vi "区域判断 - 副本.vi"(4 "压力数组":dbl[](array[numeric]), 5 "位移数组":dbl[](array[numeric]), 8 "区域最大位移":dbl, 9 "区域最小位移":dbl) -> (2 "区域最大压力":dbl=10000.0, 3 "区域最小压力":dbl)   [LabVIEW 2013]
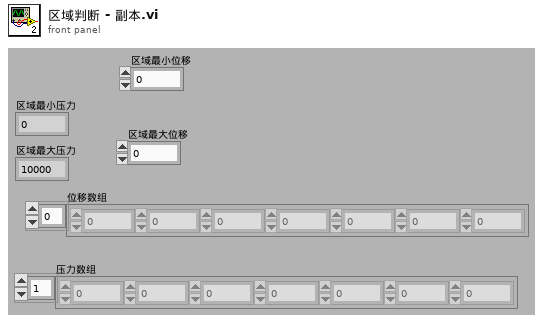
[diagram p1: front panel]
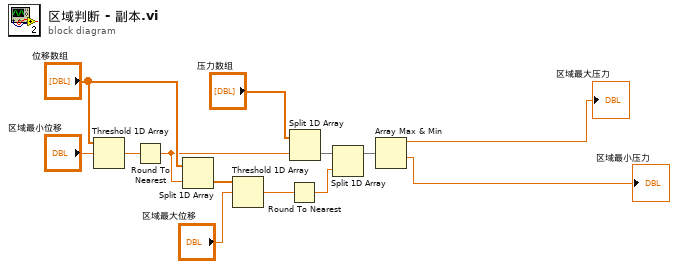
[diagram p0: block diagram]
diagram:
  n1 = Threshold 1D Array(2:"区域最小位移", 3:"位移数组") -> (0:w11:dbl)  [unwired: 1 in]
  n2 = Round To Nearest(number=w11) -> (nearest integer value=w6:dbl)
  n3 = Split 1D Array(array="位移数组", index=w6) -> (second subarray=w7:dbl[])  [unwired: 1 out]
  n4 = Threshold 1D Array(2:"区域最大位移", 3:w7) -> (0:w10:dbl)  [unwired: 1 in]
  n5 = Round To Nearest(number=w10) -> (nearest integer value=w4:dbl)
  n6 = Split 1D Array(array="压力数组", index=w6) -> (second subarray=w5:dbl[])  [unwired: 1 out]
  n7 = Split 1D Array(array=w5, index=w4) -> (first subarray=w3:dbl[])  [unwired: 1 out]
  n8 = Array Max & Min(array=w3) -> (max value=→"区域最大压力":dbl, min value=→"区域最小压力":dbl)  [unwired: 2 out]
